vi "setMode.vi"(8 "error in (no error)":errorcluster, 10 "mode":T1, 11 "DmmNiPxi in":refnum<class "DmmNi.lvclass">) -> (0 "error out":errorcluster, 3 "DmmNiPxi out":refnum<class "DmmNi.lvclass">)   [LabVIEW 2023, in "DmmNi.lvclass"]
doc: "<b>Author:</b> Wolfgang\n<b>Description:</b>Define measurement mode: Voltage, Current, Resistance"
uses:
  DmmNi.lvclass
  Data/DmmModes.ctl
  <instrlib>/niDMM/nidmm.llb/niDMM Control Actions.ctl
  DmmNi.lvclass/DmmNi.ctl
  Multimeter.lvclass
  sweDmm.lvlib
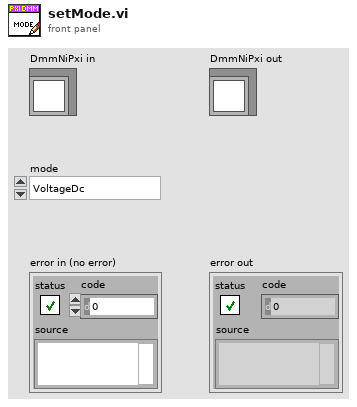
[diagram p1: front panel]
types:
  T1 = typedef "sweDmm.lvlib/DmmModes.ctl" = enum16{"VoltageDc", "VoltageAc", "CurrentDc", "CurrentAc", "Resistance2W"}
  T2 = typedef "niDMM Control Actions.ctl" = i32
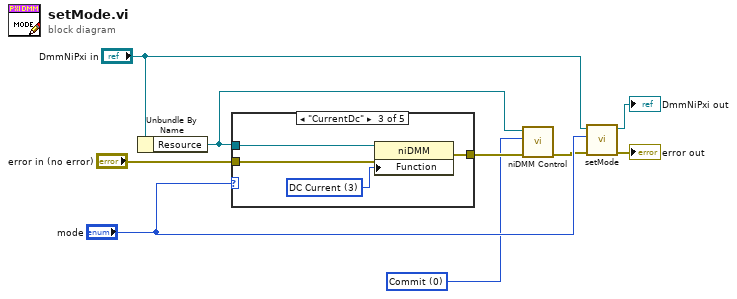
[diagram p0: block diagram]
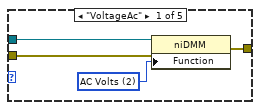
[diagram p2: hidden frame]
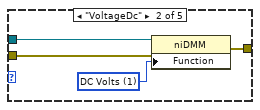
[diagram p3: hidden frame]
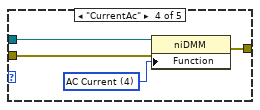
[diagram p4: hidden frame]
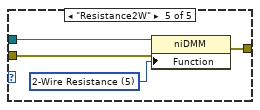
[diagram p5: hidden frame]
diagram:
  w1 = T2 0 items=["Commit"] ("Control Action")
  n1 = Unbundle By Name("DmmNiPxi in") -> ("Resource"=w2:refnum<k15>)
  n2 = case shown="\"CurrentDc\"" "mode" {
    tunnel: w2 -> [w13 w17 w21 w25 w29]
    tunnel: "error in (no error)" -> [w12 w16 w20 w24 w28]
    tunnel: [w11 w15 w19 w23 w27] -> w4
    frame "VoltageAc" {
      w10 = 2 items=["DC Volts"=1, "AC Volts"=2, "DC Current"=3, "AC Current"=4, "2-Wire Resistance"=5, "4-Wire Resistance"=101, "Frequency"=104, "Period"=105, "AC Volts DC Coupled"=1001, "Diode"=1002, "Waveform Voltage"=1003, "Waveform Current"=1004, "Capacitance"=1005, "Inductance"=1006, "Temperature"=108] ("Configuration:Function")
      n3 = property class="niDMM"(reference=w13, error in=w12, "Function"=w10) -> (error out=w11:errorcluster)  [unwired: 1 out]
    }
    frame "VoltageDc" {
      w14 = 1 items=["DC Volts"=1, "AC Volts"=2, "DC Current"=3, "AC Current"=4, "2-Wire Resistance"=5, "4-Wire Resistance"=101, "Frequency"=104, "Period"=105, "AC Volts DC Coupled"=1001, "Diode"=1002, "Waveform Voltage"=1003, "Waveform Current"=1004, "Capacitance"=1005, "Inductance"=1006, "Temperature"=108] ("Configuration:Function")
      n4 = property class="niDMM"(reference=w17, error in=w16, "Function"=w14) -> (error out=w15:errorcluster)  [unwired: 1 out]
    }
    frame "CurrentDc" {
      w18 = 3 items=["DC Volts"=1, "AC Volts"=2, "DC Current"=3, "AC Current"=4, "2-Wire Resistance"=5, "4-Wire Resistance"=101, "Frequency"=104, "Period"=105, "AC Volts DC Coupled"=1001, "Diode"=1002, "Waveform Voltage"=1003, "Waveform Current"=1004, "Capacitance"=1005, "Inductance"=1006, "Temperature"=108] ("Configuration:Function")
      n5 = property class="niDMM"(reference=w21, error in=w20, "Function"=w18) -> (error out=w19:errorcluster)  [unwired: 1 out]
    }
    frame "CurrentAc" {
      w22 = 4 items=["DC Volts"=1, "AC Volts"=2, "DC Current"=3, "AC Current"=4, "2-Wire Resistance"=5, "4-Wire Resistance"=101, "Frequency"=104, "Period"=105, "AC Volts DC Coupled"=1001, "Diode"=1002, "Waveform Voltage"=1003, "Waveform Current"=1004, "Capacitance"=1005, "Inductance"=1006, "Temperature"=108] ("Configuration:Function")
      n6 = property class="niDMM"(reference=w25, error in=w24, "Function"=w22) -> (error out=w23:errorcluster)  [unwired: 1 out]
    }
    frame "Resistance2W" {
      w26 = 5 items=["DC Volts"=1, "AC Volts"=2, "DC Current"=3, "AC Current"=4, "2-Wire Resistance"=5, "4-Wire Resistance"=101, "Frequency"=104, "Period"=105, "AC Volts DC Coupled"=1001, "Diode"=1002, "Waveform Voltage"=1003, "Waveform Current"=1004, "Capacitance"=1005, "Inductance"=1006, "Temperature"=108] ("Configuration:Function")
      n7 = property class="niDMM"(reference=w29, error in=w28, "Function"=w26) -> (error out=w27:errorcluster)  [unwired: 1 out]
    }
  }
  n8 = call <instrlib>:"niDMM Control.vi"("error in (no error)"=w4, "Control Action"=w1, "instrument handle"=w2) -> ("error out"=w3:errorcluster)  [unwired: 7 in, 1 out]
  n9 = call-parent "setMode.vi"("error in (no error)"=w3, "Mode"="mode", "Multimeter in"="DmmNiPxi in") -> ("error out"=→"error out":errorcluster, "Multimeter out"=→"DmmNiPxi out":refnum<class "DmmNi.lvclass">)  [unwired: 7 in]
